vi "Trig shutter from Raman.vi"() -> ()   [LabVIEW 2010]
uses:
  <vilib>/Waveform/DWDTOps.llb/DWDT Boolean Array to Digital.vi
panel:
  out "error out":errorcluster
  out "Numeric":i32
  out "digital waveform":digitalwaveform(waveform)={"t0"=timestamp(0 s since 1904-01-01), "dt"=0.0, "Y"={"transitions"=[], "data"=[]}, "error"={"status"=FALSE, "code"=37421928, "source"=""}}
  in  "stop (F)":bool
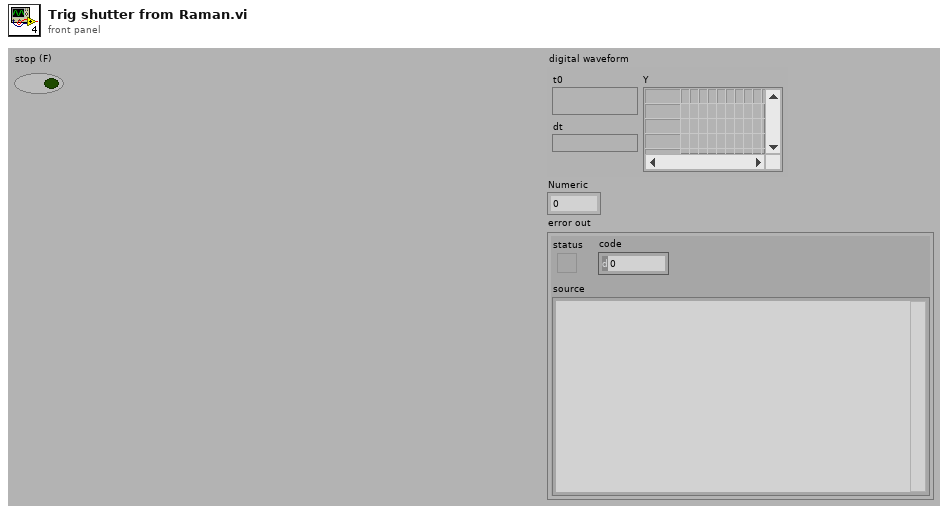
[diagram p1: front panel]
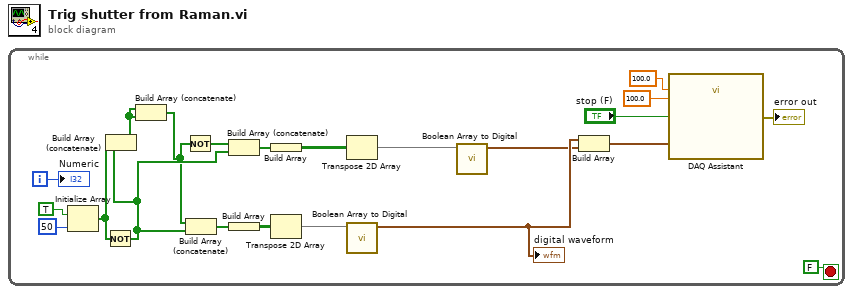
[diagram p0: block diagram]
diagram:
  n1 = while {
    i -> [w6]
    stop <- FALSE stop-if-true
    n2 = Initialize Array(TRUE, 50 ("element")) -> (w14:bool[])
    n3 = Not(x=w14) -> (.not. x?=w10:bool[])
    n4 = Build Array (concatenate)(w14, w10) -> (w4:bool[])
    n5 = Build Array (concatenate)(w4, w4) -> (w3:bool[])
    n6 = Not(x=w3) -> (.not. x?=w11:bool[])
    n7 = Build Array (concatenate)(w3, w10) -> (w13:bool[])
    n8 = Build Array (concatenate)(w11, w10) -> (w9:bool[])
    n9 = Build Array(w13) -> (w12:bool[][])
    n10 = Build Array(w9) -> (w17:bool[][])
    n11 = Transpose 2D Array(2D array=w12) -> (transposed array=w18:bool[][])
    n12 = Transpose 2D Array(2D array=w17) -> (transposed array=w16:bool[][])
    n13 = call-poly <vilib>:"Boolean Array to Digital.vi"("boolean array"=w18) -> ("digital waveform"=w2:digitalwaveform)  [unwired: 9 in, 1 out]
    "digital waveform" <- w2
    n14 = call-poly <vilib>:"Boolean Array to Digital.vi"("boolean array"=w16) -> ("digital waveform"=w1:digitalwaveform)  [unwired: 9 in, 1 out]
    n15 = Build Array(w2, w1) -> (w15:digitalwaveform[])
    n16 = call "DAQ Assistant"("data"=w15, "rate"=100.0, "timeout (s)"=100.0, "stop (T)"="stop (F)") -> ("error out"=→"error out":errorcluster)  [unwired: 14 in, 1 out]
    "Numeric" <- w6
  }
